vi "ReadSeq Test.vi"() -> ()   [LabVIEW 2016]
uses:
  Utilities/FPGA Interface/FPGA Interface.lvclass
panel:
  in  "Read":bool
  in  "Write":bool
  out "Val?":u16[](array[numeric]) format="%04x"
  in  "Val":u16[](array[numeric]) format="%04x"
  in  "Addr":u16 format="%04x"
  in  "stop":bool
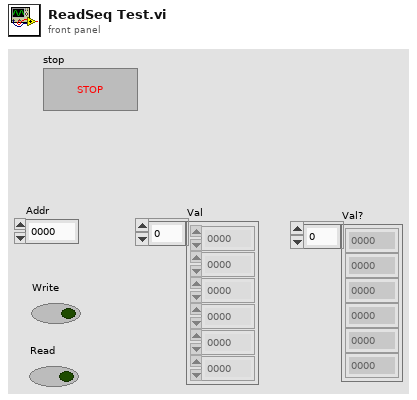
[diagram p1: front panel]
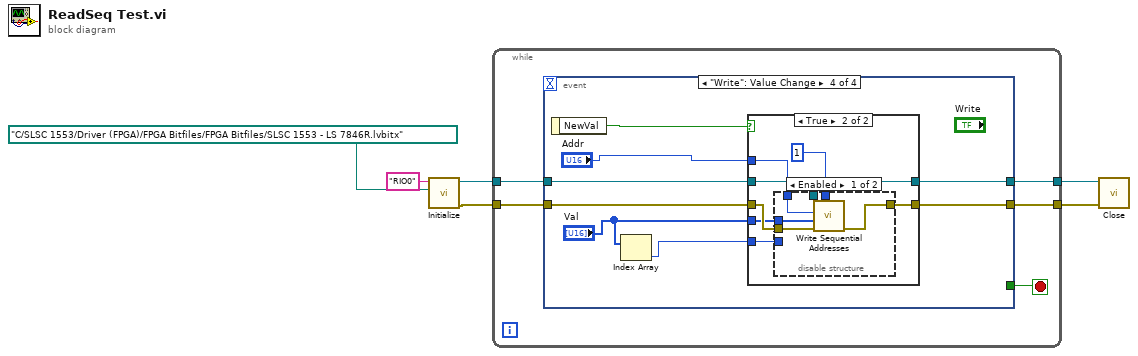
[diagram p0: block diagram]
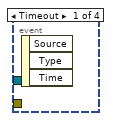
[diagram p2: hidden frame]
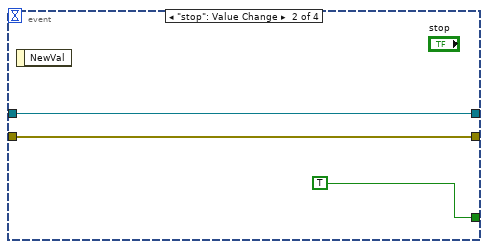
[diagram p3: hidden frame]
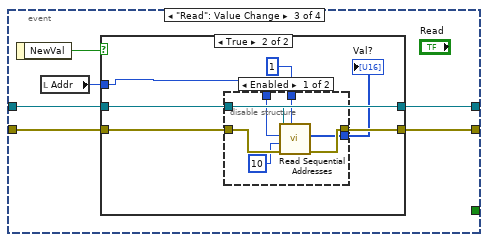
[diagram p4: hidden frame]
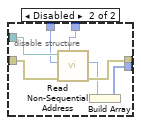
[diagram p6: hidden frame]
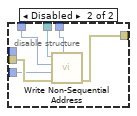
[diagram p8: hidden frame]
diagram:
  n1 = call "Initialize.vi"("Bitfile path"=path "C:/SLSC 1553/Driver (FPGA)/FPGA Bitfiles/FPGA Bitfiles/SLSC 1553 - LS 7846R.lvbitx", "Device address"="RIO0") -> ("error out"=w3:errorcluster, "FPGA Interface out"=w4:refnum<class "FPGA Interface.lvclass">)  [unwired: 8 in]
  n2 = while {
    tunnel: w4 -> [w10]
    tunnel: w3 -> [w9]
    tunnel: [w8] -> w2
    tunnel: [w7] -> w1
    stop <- w11 stop-if-true
    n3 = event shown="[3] \"Write\": Value Change" {
      selector: _ -> [_ _ _ _]
      dyn-events: _ -> [_ _ _ _]
      timeout: _ -> [_ _ _ _]
      tunnel: [_ TRUE _ _] -> w11
      tunnel: w10 -> [_ w12 w18 w48]
      tunnel: w9 -> [_ w13 w19 w49]
      tunnel: [_ w13 w17 w46] -> w8
      tunnel: [_ w12 w16 w47] -> w7
      event Timeout {
        n4 = event-data() -> ()  [unwired: 1 in, 3 out]
      }
      event "stop": Value Change {
        n5 = event-data() -> ()  [unwired: 1 in, 1 out]
      }
      event "Read": Value Change {
        n6 = event-data() -> ("NewVal"=w20:bool)  [unwired: 1 in]
        n7 = local read "Addr"() -> (w15:u16)
        n8 = case shown="True" w20 {
          tunnel: w19 -> [w22 w26]
          tunnel: w18 -> [w21 w27]
          tunnel: [w22 w25] -> w17
          tunnel: [w21 w27] -> w16
          tunnel: w15 -> [_ w23]
          frame False {
          }
          frame True {
            n9 = disable-structure shown="Enabled" {
              disable-tunnel: u8 1 ("Target IC (1-8)") -> [w35 w39]
              disable-tunnel: w27 -> [w34 w40]
              disable-tunnel: w26 -> [w33 w42]
              disable-tunnel: [w32 w41] -> w25
              disable-tunnel: [w31 w36] -> w24
              disable-tunnel: w23 -> [w30 w38]
              frame Enabled {
                n10 = call-dynamic "Read Sequential Addresses.vi"("Target IC (1-8)"=w35, "error in (no error)"=w33, "Addresses to Read"=u16 10, "Starting Address"=w30, "FPGA Interface in"=w34) -> ("error out"=w32:errorcluster, "Data"=w31:u16[])  [unwired: 5 in]
              }
              frame Disabled {
                n11 = call-dynamic "Read Non-Sequential Address.vi"("Target IC (1-8)"=w39, "error in (no error)"=w42, "Address"=w38, "FPGA Interface in"=w40) -> ("error out"=w41:errorcluster, "Data"=w37:u16)  [unwired: 6 in]
                n12 = Build Array(w37) -> (w36:u16[])
              }
            }
            "Val?" <- w24
          }
        }
      }
      event "Write": Value Change {
        n13 = event-data() -> ("NewVal"=w50:bool)  [unwired: 1 in]
        n14 = Index Array(array="Val") -> (element=w44:u16)  [unwired: 1 in]
        n15 = case shown="True" w50 {
          tunnel: [w52 w56] -> w46
          tunnel: w49 -> [w52 w58]
          tunnel: [w51 w57] -> w47
          tunnel: w48 -> [w51 w57]
          tunnel: "Addr" -> [_ w55]
          tunnel: "Val" -> [_ w54]
          tunnel: w44 -> [_ w53]
          frame False {
          }
          frame True {
            n16 = disable-structure shown="Enabled" {
              disable-tunnel: u8 1 ("Target IC (1-8)") -> [w65 w69]
              disable-tunnel: w58 -> [w64 w71]
              disable-tunnel: w57 -> [w63 w70]
              disable-tunnel: [w62 w66] -> w56
              disable-tunnel: w55 -> [w61 w68]
              disable-tunnel: w54 -> [w60 _]
              disable-tunnel: w53 -> [_ w67]
              frame Enabled {
                n17 = call-dynamic "Write Sequential Addresses.vi"("Target IC (1-8)"=w65, "error in (no error)"=w64, "Data"=w60, "Starting Address"=w61, "FPGA Interface in"=w63) -> ("error out"=w62:errorcluster)  [unwired: 6 in]
              }
              frame Disabled {
                n18 = call-dynamic "Write Non-Sequential Address.vi"("Target IC (1-8)"=w69, "error in (no error)"=w71, "Data"=w67, "Address"=w68, "FPGA Interface in"=w70) -> ("error out"=w66:errorcluster)  [unwired: 6 in]
              }
            }
          }
        }
      }
    }
  }
  n19 = call "Close.vi"("error in (no error)"=w2, "FPGA Interface in"=w1) -> ()  [unwired: 9 in, 1 out]
